vi "Get Dead Letter Source Queues.vi"(8 "error in (no error)":errorcluster, 11 "SQS in":refnum<class "NI_AWS_SQS.lvclass">) -> (0 "error out":errorcluster, 2 "Dead Letter Source Queue URLs":string[](array[string]), 3 "SQS out":refnum<class "NI_AWS_SQS.lvclass">)   [LabVIEW 2015, in "NI_AWS_SQS.lvclass"]
uses:
  NI_AWS_SQS.lvclass
  Core/Name Value Pair.ctl
  Core/Request Options.ctl
  NI_AWS_SQS.lvclass/NI_AWS_SQS.ctl
  Read Account Number.vi
  Read Name.vi
  Core/NI_AWS_Core.lvclass
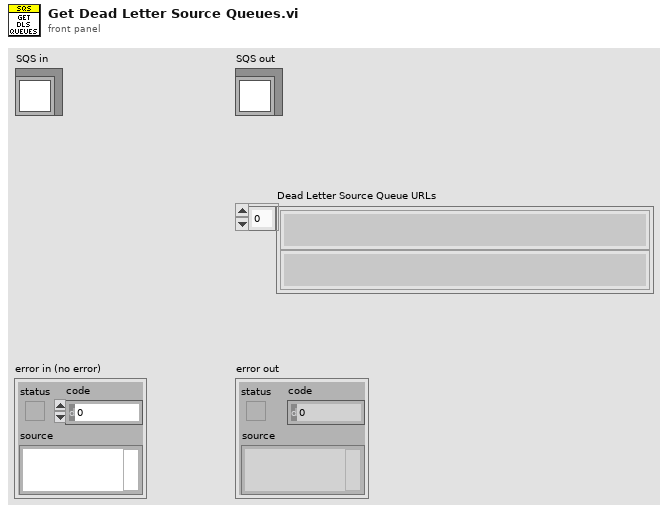
[diagram p1: front panel]
types:
  T1 = typedef "NI_AWS_Core.lvclass/Request Options.ctl" = cluster{"request headers":T2[], "request parameters":T2[], "request body":string}
  T2 = typedef "NI_AWS_Core.lvclass/Name Value Pair.ctl" = cluster{"name":string, "value":string}
  T3 = typedef "NI_AWS_Core.lvclass/Response.ctl" = cluster{"Headers":string, "Body":string}
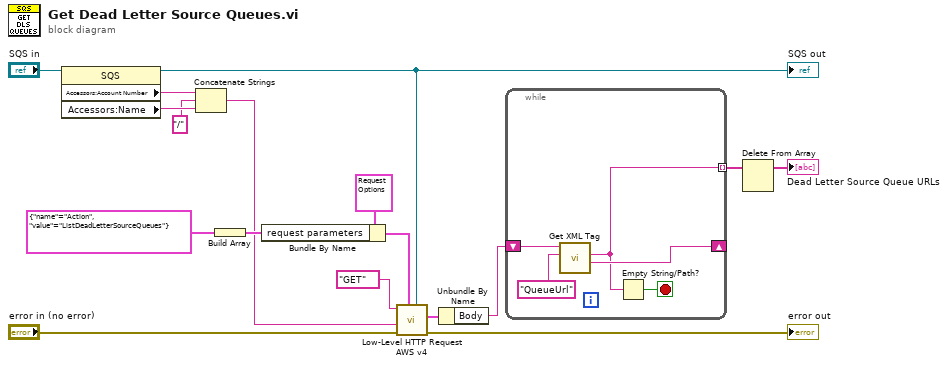
[diagram p0: block diagram]
diagram:
  n1 = property class="SQS"(reference="SQS in") -> (reference out=w6:refnum<class "NI_AWS_SQS.lvclass">, "Accessors:Account Number"=w5:string, "Accessors:Name"=w4:string)  [unwired: 1 in, 1 out]
  "SQS out" <- w6
  n2 = Concatenate Strings(w5, "/", w4) -> (w2:string)
  n3 = Build Array(T2 {"name"="Action", "value"="ListDeadLetterSourceQueues"} ("Cluster")) -> (w7:T2[])
  n4 = Bundle By Name(cluster=T1 {"request headers"=[], "request parameters"=[{"name"="Action", "value"="ListQueues"}], "request body"=""} ("Request Options"), "request parameters"=w7) -> (w8:T1)
  n5 = call "Low-Level HTTP Request AWS v4.vi"("AWS Core"=w6, "Request Options"=w8, "error in (no error)"="error in (no error)", "URL Suffix"=w2, "HTTP-Verb"="GET") -> ("error out"=→"error out":errorcluster, "Response"=w13:T3)  [unwired: 4 in, 1 out]
  n6 = Unbundle By Name(w13) -> ("Body"=w12:string)
  n7 = while {
    shift-right: [w21] -> _
    shift-left: w12 -> [w22]
    tunnel: [w18] -> w11 mode=indexing
    stop <- w20 stop-if-true
    n8 = call "Get XML Tag.vi"("Tag name"="QueueUrl", "XML String in"=w22) -> ("Remaining string"=w21:string, "Tag value"=w18:string)  [unwired: 5 in, 3 out]
    n9 = Empty String/Path?(string/path=w18) -> (empty?=w20:bool)
  }
  n10 = Delete From Array(array=w11) -> (array with subset deleted=→"Dead Letter Source Queue URLs":string[])  [unwired: 2 in, 1 out]
